vi "test - Datetype Check.vi"(8 "error in (no error)":errorcluster, 11 "TestCase in":refnum<class "testcase-Supported-Datatype.lvclass">) -> (0 "error out":errorcluster, 3 "TestCase out":refnum<class "testcase-Supported-Datatype.lvclass">)   [LabVIEW 2017, in "testcase-Supported-Datatype.lvclass"]
uses:
  testcase-Supported-Datatype.lvclass
  <vilib>/addons/_JKI Toolkits/VI Tester/TestCase.llb/TestCase.lvclass
  API-String-Arugments-Support/API String Arguments Support.lvlib
  C:/Program Files (x86)/National Instruments/LabVIEW 2017/vi.lib/addons/_JKI Toolkits/VI Tester/TestCase.llb/TestCase.lvclass
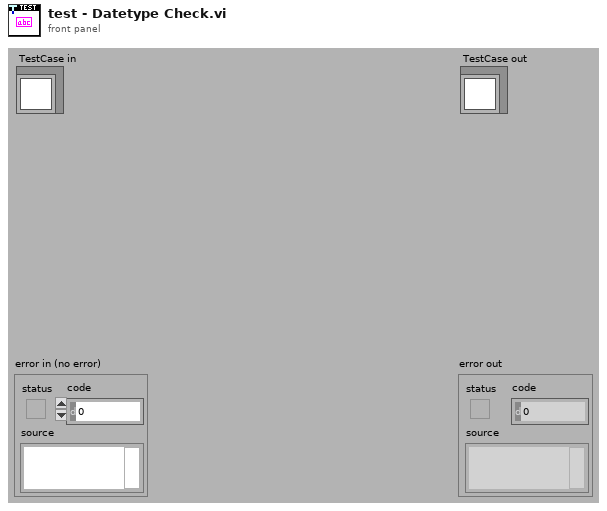
[diagram p1: front panel]
types:
  T1 = cluster{"Name":string, "Child":cluster{"Name":string}, "Bool":bool}[]
  T2 = cluster{"Name":string, "Child":cluster{"Name":string}, "Bool":bool}
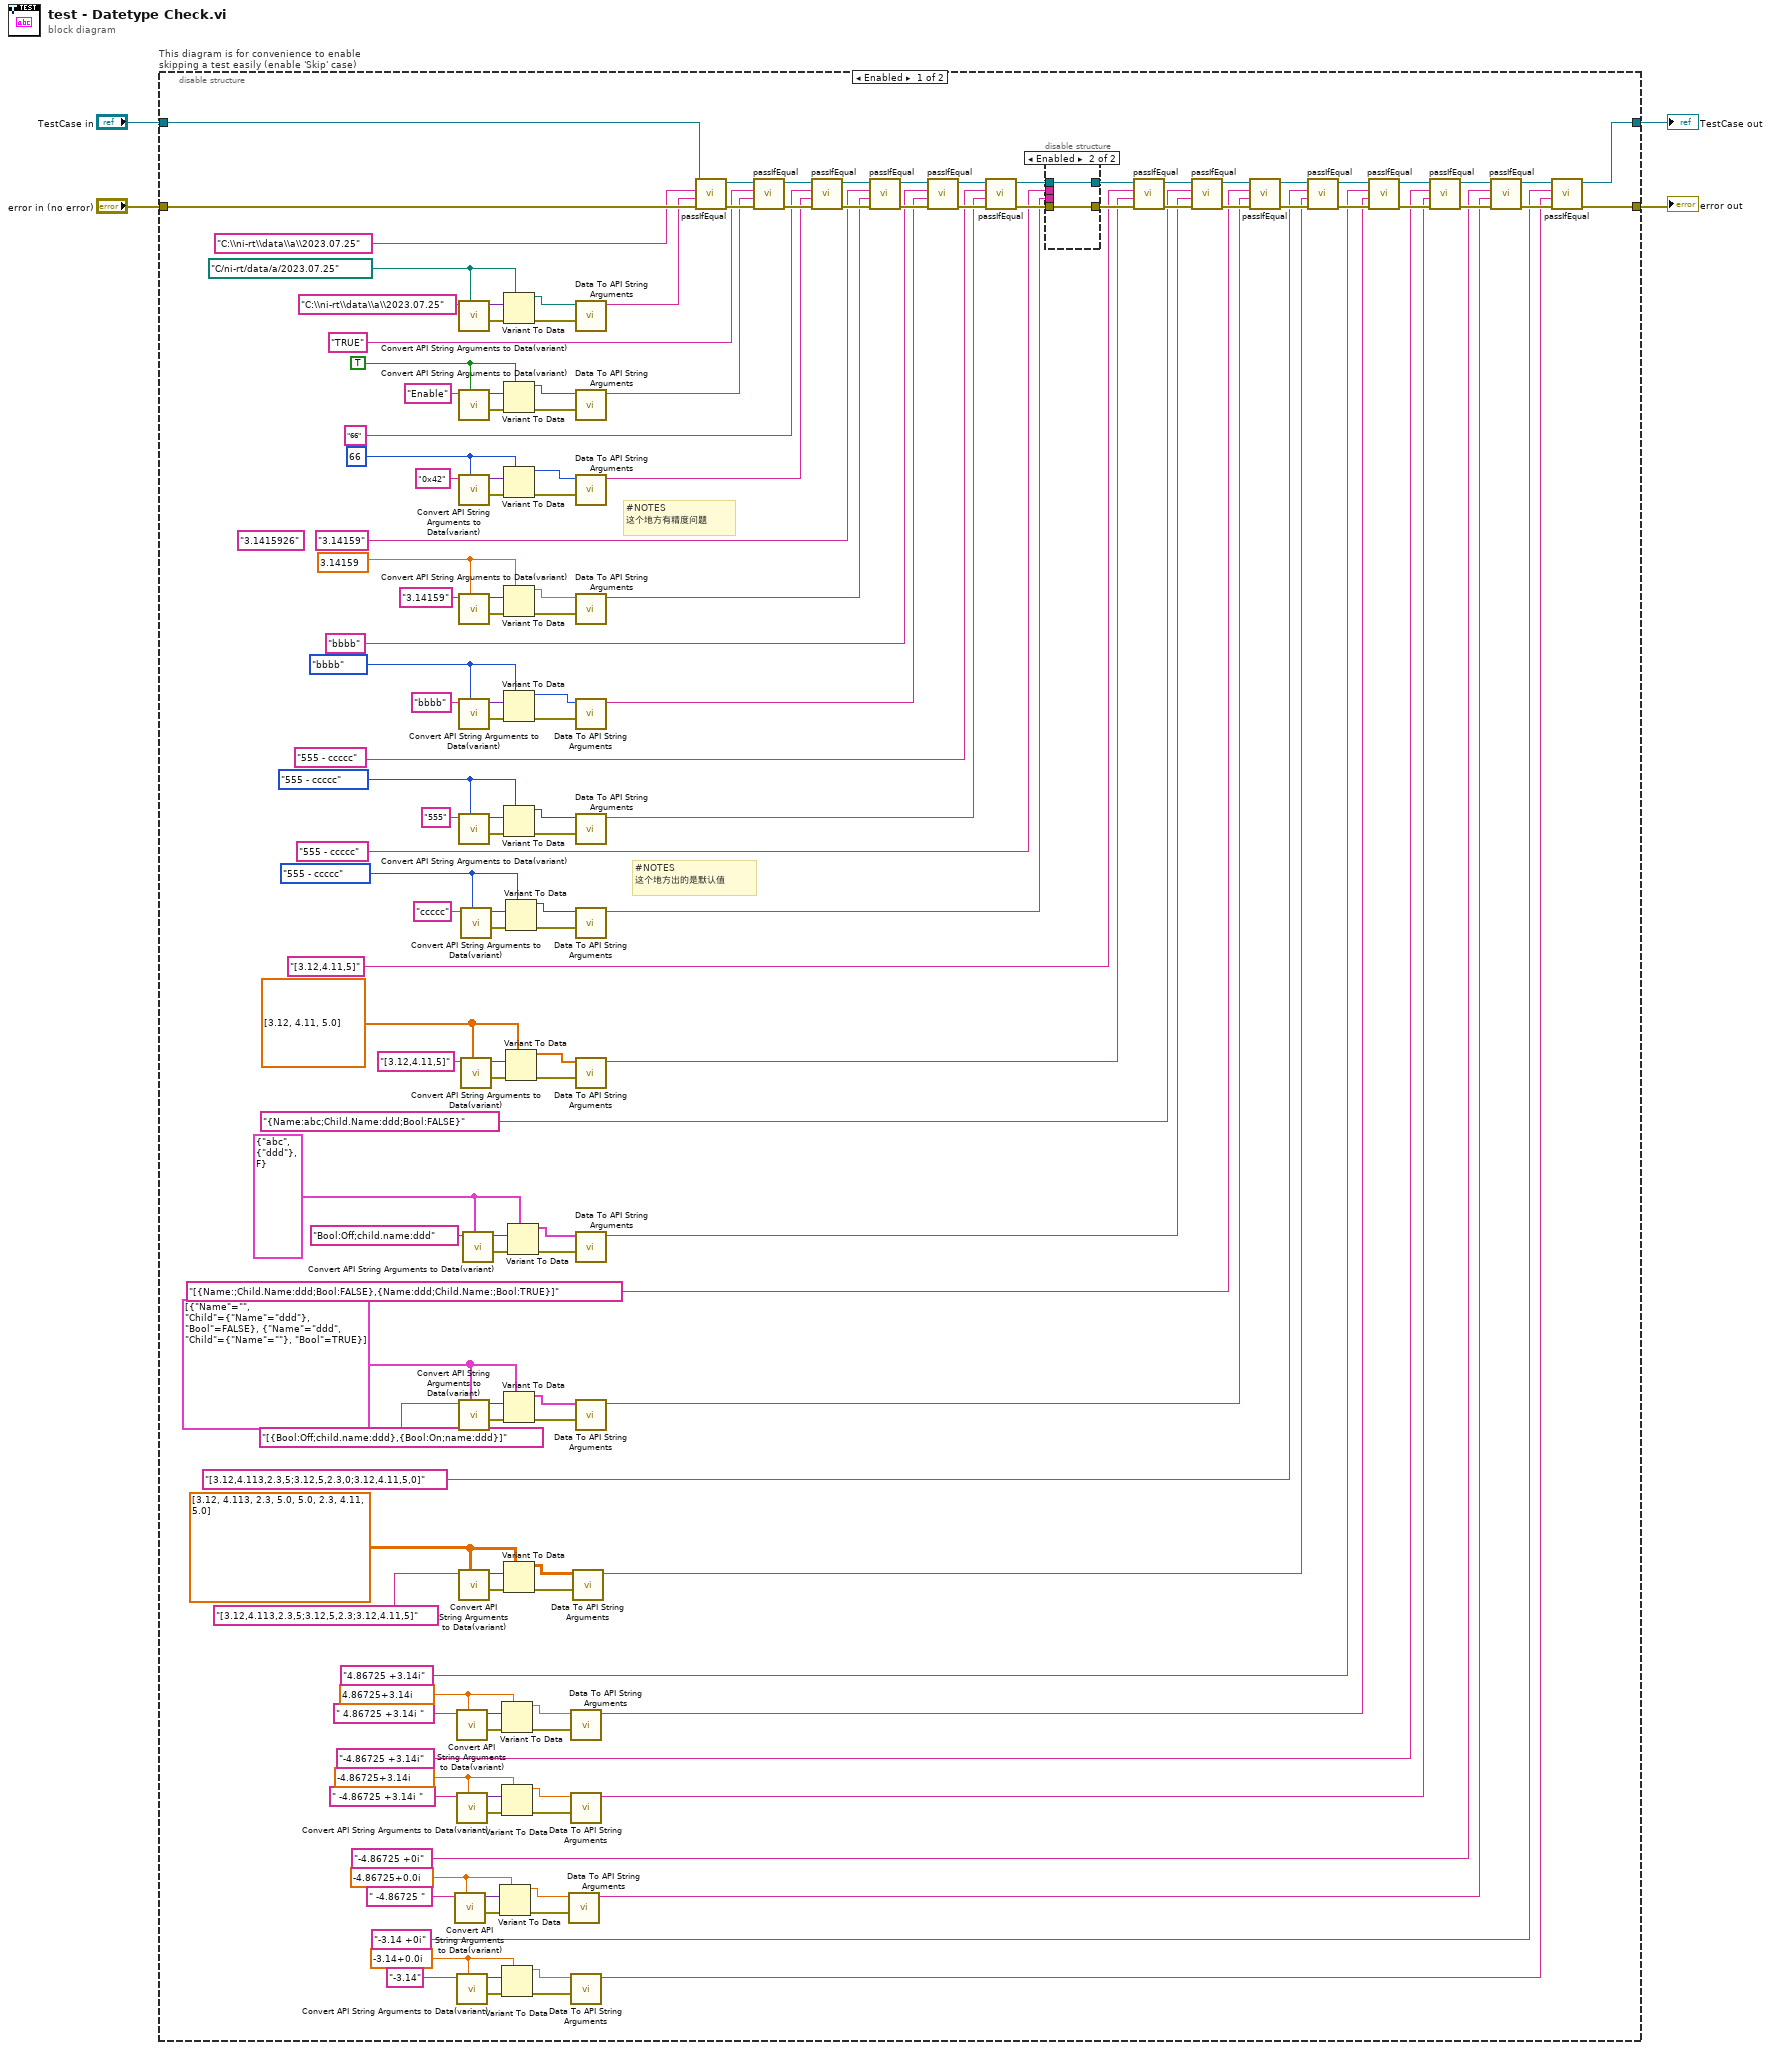
[diagram p0: block diagram]
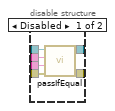
[diagram p2: hidden frame]
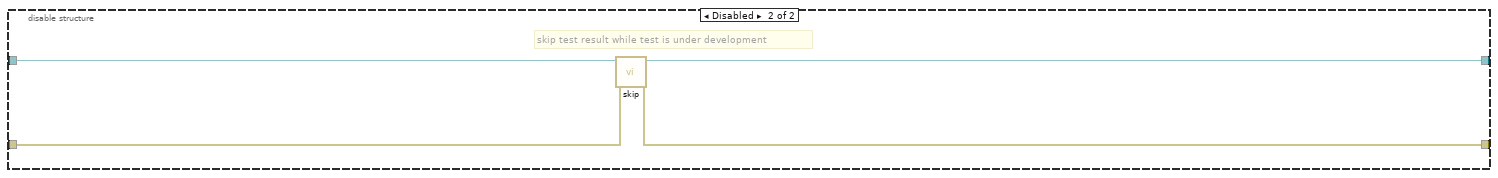
[diagram p3: hidden frame]
diagram:
  n1 = disable-structure "This diagram is for convenience to enable skipping a test easily (enable 'Skip' case)" shown="Enabled" {
    disable-tunnel: "TestCase in" -> [w156 w168]
    disable-tunnel: [w32 w166] -> w1
    disable-tunnel: [w31 w167] -> w3
    disable-tunnel: "error in (no error)" -> [w155 w165]
    frame Enabled {
      w11 = cdb -3.14+0.0i ("Data 14")
      w13 = cdb -4.86725+0.0i ("Data 15")
      w15 = cdb -4.86725+3.14i ("Data 13")
      w41 = cdb 4.86725+3.14i ("Data 12")
      w72 = enum16{"1 - aaaa", "2 - bbbb", "555 - ccccc"}."555 - ccccc" ("Data 6")
      (unwired) "3.1415926" ("String 21")
      w99 = dbl[][] [[3.12, 4.113, 2.3, 5.0, 5.0, 2.3, 4.11, 5.0]] ("Data 11")
      w105 = T1 [{"Name"="", "Child"={"Name"="ddd"}, "Bool"=FALSE}, {"Name"="ddd", "Child"={"Name"=""}, "Bool"=TRUE}] ("Data 10")
      w111 = T2 {"Name"="abc", "Child"={"Name"="ddd"}, "Bool"=FALSE} ("Data 8")
      w117 = dbl[] [3.12, 4.11, 5.0] ("Data 4")
      w123 = enum16{"1 - aaaa", "2 - bbbb", "555 - ccccc"}."555 - ccccc" ("Data 6")
      w129 = enum16{"aaaa", "bbbb", "ccccc"}."bbbb" ("Data 5")
      w133 = 3.14159
      w139 = 66
      w92 = TRUE
      w151 = path "C:/ni-rt/data/a/2023.07.25" ("Data 9")
      # "#NOTES\n这个地方出的是默认值"
      # "#NOTES\n这个地方有精度问题"
      n2 = call "Convert API String Arguments to Data(variant).vi"("Type"=w13, "String"=" -4.86725 " ("String 32")) -> ("error"=w22:errorcluster, "Data"=w21:variant)  [unwired: 8 in]
      n3 = call "Convert API String Arguments to Data(variant).vi"("Type"=w41, "String"=" 4.86725 +3.14i " ("String 26")) -> ("error"=w44:errorcluster, "Data"=w43:variant)  [unwired: 8 in]
      n4 = call "Convert API String Arguments to Data(variant).vi"("Type"=w15, "String"=" -4.86725 +3.14i " ("String 28")) -> ("error"=w27:errorcluster, "Data"=w28:variant)  [unwired: 8 in]
      n5 = call "Convert API String Arguments to Data(variant).vi"("Type"=w11, "String"="-3.14" ("String 30")) -> ("error"=w19:errorcluster, "Data"=w20:variant)  [unwired: 8 in]
      n6 = call "Convert API String Arguments to Data(variant).vi"("Type"=w151, "String"="C:\\ni-rt\\data\\a\\2023.07.25") -> ("error"=w154:errorcluster, "Data"=w153:variant)  [unwired: 8 in]
      n7 = call "Convert API String Arguments to Data(variant).vi"("Type"=w92, "String"="Enable") -> ("error"=w149:errorcluster, "Data"=w148:variant)  [unwired: 8 in]
      n8 = call "Convert API String Arguments to Data(variant).vi"("Type"=w139, "String"="0x42") -> ("error"=w142:errorcluster, "Data"=w143:variant)  [unwired: 8 in]
      n9 = call "Convert API String Arguments to Data(variant).vi"("Type"=w133, "String"="3.14159") -> ("error"=w138:errorcluster, "Data"=w137:variant)  [unwired: 8 in]
      n10 = call "Convert API String Arguments to Data(variant).vi"("Type"=w129, "String"="bbbb") -> ("error"=w132:errorcluster, "Data"=w131:variant)  [unwired: 8 in]
      n11 = call "Convert API String Arguments to Data(variant).vi"("Type"=w123, "String"="555") -> ("error"=w124:errorcluster, "Data"=w125:variant)  [unwired: 8 in]
      n12 = call "Convert API String Arguments to Data(variant).vi"("Type"=w105, "String"="[{Bool:Off;child.name:ddd},{Bool:On;name:ddd}]") -> ("error"=w110:errorcluster, "Data"=w109:variant)  [unwired: 8 in]
      n13 = call "Convert API String Arguments to Data(variant).vi"("Type"=w99, "String"="[3.12,4.113,2.3,5;3.12,5,2.3;3.12,4.11,5]") -> ("error"=w102:errorcluster, "Data"=w103:variant)  [unwired: 8 in]
      n14 = call "Convert API String Arguments to Data(variant).vi"("Type"=w72, "String"="ccccc") -> ("error"=w71:errorcluster, "Data"=w70:variant)  [unwired: 8 in]
      n15 = call "Convert API String Arguments to Data(variant).vi"("Type"=w117, "String"="[3.12,4.11,5]") -> ("error"=w120:errorcluster, "Data"=w119:variant)  [unwired: 8 in]
      n16 = call "Convert API String Arguments to Data(variant).vi"("Type"=w111, "String"="Bool:Off;child.name:ddd") -> ("error"=w114:errorcluster, "Data"=w115:variant)  [unwired: 8 in]
      n17 = Variant To Data(error in=w22, type=w13, Variant=w21) -> (data=w24:cdb, error out=w23:errorcluster)
      n18 = Variant To Data(error in=w44, type=w41, Variant=w43) -> (data=w46:cdb, error out=w45:errorcluster)
      n19 = Variant To Data(error in=w27, type=w15, Variant=w28) -> (data=w25:cdb, error out=w26:errorcluster)
      n20 = Variant To Data(error in=w19, type=w11, Variant=w20) -> (data=w17:cdb, error out=w18:errorcluster)
      n21 = Variant To Data(error in=w154, type=w151, Variant=w153) -> (data=w97:path, error out=w98:errorcluster)
      n22 = Variant To Data(error in=w149, type=w92, Variant=w148) -> (data=w95:bool, error out=w94:errorcluster)
      n23 = Variant To Data(error in=w142, type=w139, Variant=w143) -> (data=w89:i32, error out=w90:errorcluster)
      n24 = Variant To Data(error in=w138, type=w133, Variant=w137) -> (data=w85:dbl, error out=w86:errorcluster)
      n25 = Variant To Data(error in=w132, type=w129, Variant=w131) -> (data=w81:enum16{"aaaa", "bbbb", "ccccc"}, error out=w82:errorcluster)
      n26 = Variant To Data(error in=w124, type=w123, Variant=w125) -> (data=w76:enum16{"1 - aaaa", "2 - bbbb", "555 - ccccc"}, error out=w77:errorcluster)
      n27 = Variant To Data(error in=w110, type=w105, Variant=w109) -> (data=w53:T1, error out=w54:errorcluster)
      n28 = Variant To Data(error in=w102, type=w99, Variant=w103) -> (data=w49:dbl[][], error out=w50:errorcluster)
      n29 = Variant To Data(error in=w71, type=w72, Variant=w70) -> (data=w74:enum16{"1 - aaaa", "2 - bbbb", "555 - ccccc"}, error out=w73:errorcluster)
      n30 = Variant To Data(error in=w120, type=w117, Variant=w119) -> (data=w61:dbl[], error out=w62:errorcluster)
      n31 = Variant To Data(error in=w114, type=w111, Variant=w115) -> (data=w57:T2, error out=w58:errorcluster)
      n32 = call "Data To API String Arguments.vi"("error in (no error)"=w23, "data"=w24) -> ("String"=w7:string)  [unwired: 8 in, 1 out]
      n33 = call "Data To API String Arguments.vi"("error in (no error)"=w45, "data"=w46) -> ("String"=w30:string)  [unwired: 8 in, 1 out]
      n34 = call "Data To API String Arguments.vi"("error in (no error)"=w26, "data"=w25) -> ("String"=w9:string)  [unwired: 8 in, 1 out]
      n35 = call "Data To API String Arguments.vi"("error in (no error)"=w18, "data"=w17) -> ("String"=w5:string)  [unwired: 8 in, 1 out]
      n36 = call "Data To API String Arguments.vi"("error in (no error)"=w50, "data"=w49) -> ("String"=w48:string)  [unwired: 8 in, 1 out]
      n37 = call "Data To API String Arguments.vi"("error in (no error)"=w98, "data"=w97) -> ("String"=w96:string)  [unwired: 8 in, 1 out]
      n38 = call "Data To API String Arguments.vi"("error in (no error)"=w94, "data"=w95) -> ("String"=w91:string)  [unwired: 8 in, 1 out]
      n39 = call "Data To API String Arguments.vi"("error in (no error)"=w90, "data"=w89) -> ("String"=w88:string)  [unwired: 8 in, 1 out]
      n40 = call "Data To API String Arguments.vi"("error in (no error)"=w86, "data"=w85) -> ("String"=w84:string)  [unwired: 8 in, 1 out]
      n41 = call "Data To API String Arguments.vi"("error in (no error)"=w82, "data"=w81) -> ("String"=w80:string)  [unwired: 8 in, 1 out]
      n42 = call "Data To API String Arguments.vi"("error in (no error)"=w77, "data"=w76) -> ("String"=w75:string)  [unwired: 8 in, 1 out]
      n43 = call "Data To API String Arguments.vi"("error in (no error)"=w73, "data"=w74) -> ("String"=w63:string)  [unwired: 8 in, 1 out]
      n44 = call "Data To API String Arguments.vi"("error in (no error)"=w62, "data"=w61) -> ("String"=w60:string)  [unwired: 8 in, 1 out]
      n45 = call "Data To API String Arguments.vi"("error in (no error)"=w58, "data"=w57) -> ("String"=w56:string)  [unwired: 8 in, 1 out]
      n46 = call "Data To API String Arguments.vi"("error in (no error)"=w54, "data"=w53) -> ("String"=w52:string)  [unwired: 8 in, 1 out]
      n47 = call-dynamic "passIfEqual.vi"("error in (no error)"=w155, "y"=w96, "x"="C:\\ni-rt\\data\\a\\2023.07.25" ("String 10"), "TestCase in"=w156) -> ("error out"=w146:errorcluster, "TestCase out"=w145:refnum<class "testcase-Supported-Datatype.lvclass">)  [unwired: 6 in]
      n48 = call-dynamic "passIfEqual.vi"("error in (no error)"=w146, "y"=w91, "x"="TRUE" ("String 23"), "TestCase in"=w145) -> ("error out"=w141:errorcluster, "TestCase out"=w140:refnum<class "testcase-Supported-Datatype.lvclass">)  [unwired: 6 in]
      n49 = call-dynamic "passIfEqual.vi"("error in (no error)"=w141, "y"=w88, "x"="66" ("String 22"), "TestCase in"=w140) -> ("error out"=w134:errorcluster, "TestCase out"=w135:refnum<class "testcase-Supported-Datatype.lvclass">)  [unwired: 6 in]
      n50 = call-dynamic "passIfEqual.vi"("error in (no error)"=w134, "y"=w84, "x"="3.14159" ("String 21"), "TestCase in"=w135) -> ("error out"=w128:errorcluster, "TestCase out"=w127:refnum<class "testcase-Supported-Datatype.lvclass">)  [unwired: 6 in]
      n51 = call-dynamic "passIfEqual.vi"("error in (no error)"=w128, "y"=w80, "x"="bbbb" ("String 20"), "TestCase in"=w127) -> ("error out"=w122:errorcluster, "TestCase out"=w121:refnum<class "testcase-Supported-Datatype.lvclass">)  [unwired: 6 in]
      n52 = call-dynamic "passIfEqual.vi"("error in (no error)"=w122, "y"=w75, "x"="555 - ccccc" ("String 19"), "TestCase in"=w121) -> ("error out"=w66:errorcluster, "TestCase out"=w68:refnum<class "testcase-Supported-Datatype.lvclass">)  [unwired: 6 in]
      n53 = disable-structure shown="Enabled" {
        disable-tunnel: w68 -> [w162 w164]
        disable-tunnel: [w161 w164] -> w67
        disable-tunnel: w66 -> [w160 w163]
        disable-tunnel: [w159 w163] -> w65
        disable-tunnel: "555 - ccccc" ("String 19") -> [w158 _]
        disable-tunnel: w63 -> [w157 _]
        frame Disabled {
          n54 = call-dynamic "passIfEqual.vi"("error in (no error)"=w160, "y"=w157, "x"=w158, "TestCase in"=w162) -> ("error out"=w159:errorcluster, "TestCase out"=w161:refnum<class "testcase-Supported-Datatype.lvclass">)  [unwired: 6 in]
        }
        frame Enabled {
        }
      }
      n55 = call-dynamic "passIfEqual.vi"("error in (no error)"=w65, "y"=w60, "x"="[3.12,4.11,5]" ("String 17"), "TestCase in"=w67) -> ("error out"=w112:errorcluster, "TestCase out"=w113:refnum<class "testcase-Supported-Datatype.lvclass">)  [unwired: 6 in]
      n56 = call-dynamic "passIfEqual.vi"("error in (no error)"=w112, "y"=w56, "x"="{Name:abc;Child.Name:ddd;Bool:FALSE}" ("String 16"), "TestCase in"=w113) -> ("error out"=w106:errorcluster, "TestCase out"=w107:refnum<class "testcase-Supported-Datatype.lvclass">)  [unwired: 6 in]
      n57 = call-dynamic "passIfEqual.vi"("error in (no error)"=w106, "y"=w52, "x"="[{Name:;Child.Name:ddd;Bool:FALSE},{Name:ddd;Child.Name:;Bool:TRUE}]" ("String"), "TestCase in"=w107) -> ("error out"=w100:errorcluster, "TestCase out"=w101:refnum<class "testcase-Supported-Datatype.lvclass">)  [unwired: 6 in]
      n58 = call-dynamic "passIfEqual.vi"("error in (no error)"=w100, "y"=w48, "x"="[3.12,4.113,2.3,5;3.12,5,2.3,0;3.12,4.11,5,0]" ("String 13"), "TestCase in"=w101) -> ("error out"=w39:errorcluster, "TestCase out"=w40:refnum<class "testcase-Supported-Datatype.lvclass">)  [unwired: 6 in]
      n59 = call-dynamic "passIfEqual.vi"("error in (no error)"=w39, "y"=w30, "x"="4.86725 +3.14i" ("String 25"), "TestCase in"=w40) -> ("error out"=w37:errorcluster, "TestCase out"=w38:refnum<class "testcase-Supported-Datatype.lvclass">)  [unwired: 6 in]
      n60 = call-dynamic "passIfEqual.vi"("error in (no error)"=w37, "y"=w9, "x"="-4.86725 +3.14i" ("String 27"), "TestCase in"=w38) -> ("error out"=w35:errorcluster, "TestCase out"=w36:refnum<class "testcase-Supported-Datatype.lvclass">)  [unwired: 6 in]
      n61 = call-dynamic "passIfEqual.vi"("error in (no error)"=w35, "y"=w7, "x"="-4.86725 +0i" ("String 31"), "TestCase in"=w36) -> ("error out"=w33:errorcluster, "TestCase out"=w34:refnum<class "testcase-Supported-Datatype.lvclass">)  [unwired: 6 in]
      n62 = call-dynamic "passIfEqual.vi"("error in (no error)"=w33, "y"=w5, "x"="-3.14 +0i" ("String 29"), "TestCase in"=w34) -> ("error out"=w31:errorcluster, "TestCase out"=w32:refnum<class "testcase-Supported-Datatype.lvclass">)  [unwired: 6 in]
    }
    frame Disabled {
      # "skip test result while test is under development"
      n63 = call <vilib>:"skip.vi"("error in (no error)"=w165, "TestCase in"=w168) -> ("error out"=w167:errorcluster, "TestCase out"=w166:refnum<class "testcase-Supported-Datatype.lvclass">)  [unwired: 8 in]
    }
  }
  "error out" <- w3
  "TestCase out" <- w1
